vi "PZT_Move_Buttons (SubVI).vi"(4 "PZTZ-":bool, 6 "PZTZ+":bool, 7 "PZTX+":bool, 9 "PZTY-":bool, 10 "PZTY+":bool, 11 "PZTX-":bool) -> (3 "Array":dbl[](array[numeric]))   [LabVIEW 2016]
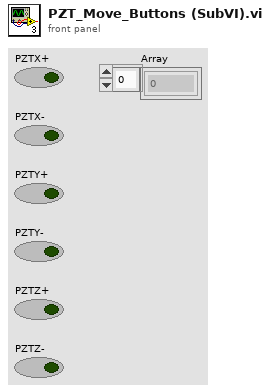
[diagram p1: front panel]
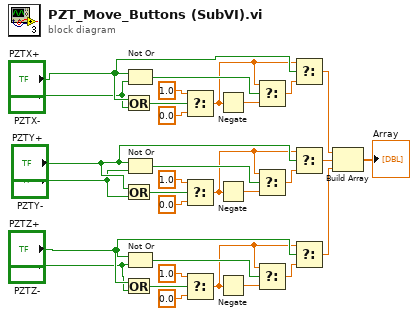
[diagram p0: block diagram]
diagram:
  n1 = Or(x="PZTX+", y="PZTX-") -> (x .or. y?=w12:bool)
  n2 = Or(x="PZTY+", y="PZTY-") -> (x .or. y?=w9:bool)
  n3 = Or(x="PZTZ+", y="PZTZ-") -> (x .or. y?=w6:bool)
  n4 = Not Or(1:"PZTX-", 2:"PZTX+") -> (0:w25:bool)
  n5 = Not Or(1:"PZTY-", 2:"PZTY+") -> (0:w26:bool)
  n6 = Not Or(1:"PZTZ-", 2:"PZTZ+") -> (0:w27:bool)
  n7 = Select(t=1.0, s=w12, f=0.0) -> (s? t:f=w13:dbl)
  n8 = Select(t=1.0, s=w9, f=0.0) -> (s? t:f=w17:dbl)
  n9 = Select(t=1.0, s=w6, f=0.0) -> (s? t:f=w20:dbl)
  n10 = Negate(x=w13) -> (-x=w14:dbl)
  n11 = Negate(x=w17) -> (-x=w18:dbl)
  n12 = Negate(x=w20) -> (-x=w21:dbl)
  n13 = Select(t=w13, s=w25, f=w14) -> (s? t:f=w15:dbl)
  n14 = Select(t=w17, s=w26, f=w18) -> (s? t:f=w16:dbl)
  n15 = Select(t=w20, s=w27, f=w21) -> (s? t:f=w19:dbl)
  n16 = Select(t=w13, s="PZTX+", f=w15) -> (s? t:f=w3:dbl)
  n17 = Select(t=w17, s="PZTY+", f=w16) -> (s? t:f=w2:dbl)
  n18 = Select(t=w20, s="PZTZ+", f=w19) -> (s? t:f=w1:dbl)
  n19 = Build Array(w3, w2, w1) -> (→"Array":dbl[])
